vi "WW_Course_Wool_Parameter.vi"() -> (0 "strValveControlState":T1, 1 "strWaterLevel":T2, 2 "strTurnOnOff":T3, 3 "strAllTime":T4, 4 "mu16ArrayBubbleSoakState":u16[](array[numeric]), 5 "mu16ArrayHeating":u16[][](array[numeric]))   [LabVIEW 2011]
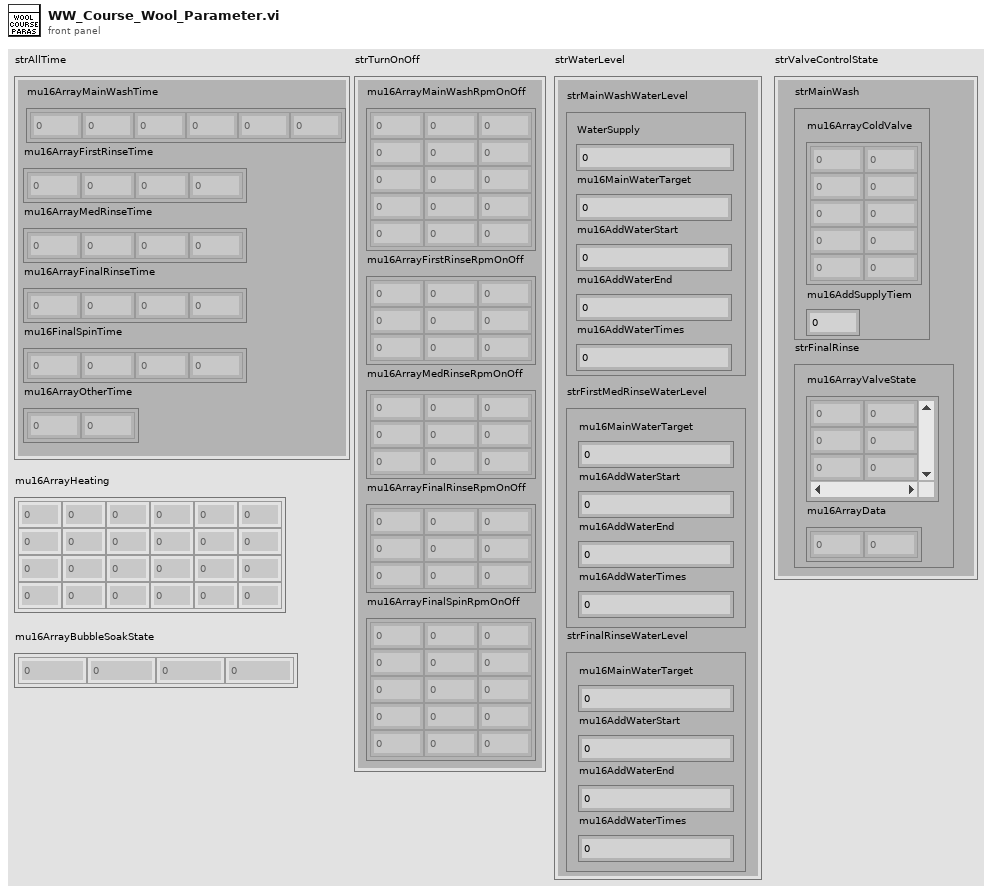
[diagram p1: front panel]
types:
  T1 = cluster{"strMainWash":cluster{"mu16ArrayColdValve":u8[][], "mu16AddSupplyTiem":u8}, "strFinalRinse":cluster{"mu16ArrayValveState":u8[][], "mu16ArrayData":u8[]}}
  T2 = cluster{"strMainWashWaterLevel":cluster{"WaterSupply":u16, "mu16MainWaterTarget":u16, "mu16AddWaterStart":u16, "mu16AddWaterEnd":u16, "mu16AddWaterTimes":u16}, "strFirstMedRinseWaterLevel":cluster{"mu16MainWaterTarget":u16, "mu16AddWaterStart":u16, "mu16AddWaterEnd":u16, "mu16AddWaterTimes":u16}, "strFinalRinseWaterLevel":cluster{"mu16MainWaterTarget":u16, "mu16AddWaterStart":u16, "mu16AddWaterEnd":u16, "mu16AddWaterTimes":u16}}
  T3 = cluster{"mu16ArrayMainWashRpmOnOff":u8[][], "mu16ArrayFirstRinseRpmOnOff":u8[][], "mu16ArrayMedRinseRpmOnOff":u8[][], "mu16ArrayFinalRinseRpmOnOff":u8[][], "mu16ArrayFinalSpinRpmOnOff":u16[][]}
  T4 = cluster{"mu16ArrayMainWashTime":u16[], "mu16ArrayFirstRinseTime":u16[], "mu16ArrayMedRinseTime":u16[], "mu16ArrayFinalRinseTime":u16[], "mu16FinalSpinTime":u16[], "mu16ArrayOtherTime":u16[]}
  T5 = enum8{"NULL", "Course", "eCotton", "Synthetics", "Wool", "Spin", "RinseSpin", "EcoDrumClean", "DarkGarment", "OutDoorCare", "BabyCare", "Delicates", "Bedding", "SuperEcoWash", "SuperSpeed"}
  T6 = cluster{"数组":u16[], "数组":u16[], "数组":u16[], "数组":u16[], "数组":u16[], "数组":u16[]}
  T7 = cluster{i32[][], i32[][], i32[][], i32[][], i32[][]}
  T8 = cluster{cluster{i32, i32, i32, i32, i32}, cluster{i32, i32, i32, i32}, cluster{"offset past number":i32, i32, i32, i32}}
  T9 = cluster{cluster{i32[][], i32}, cluster{i32[][], i32[]}}
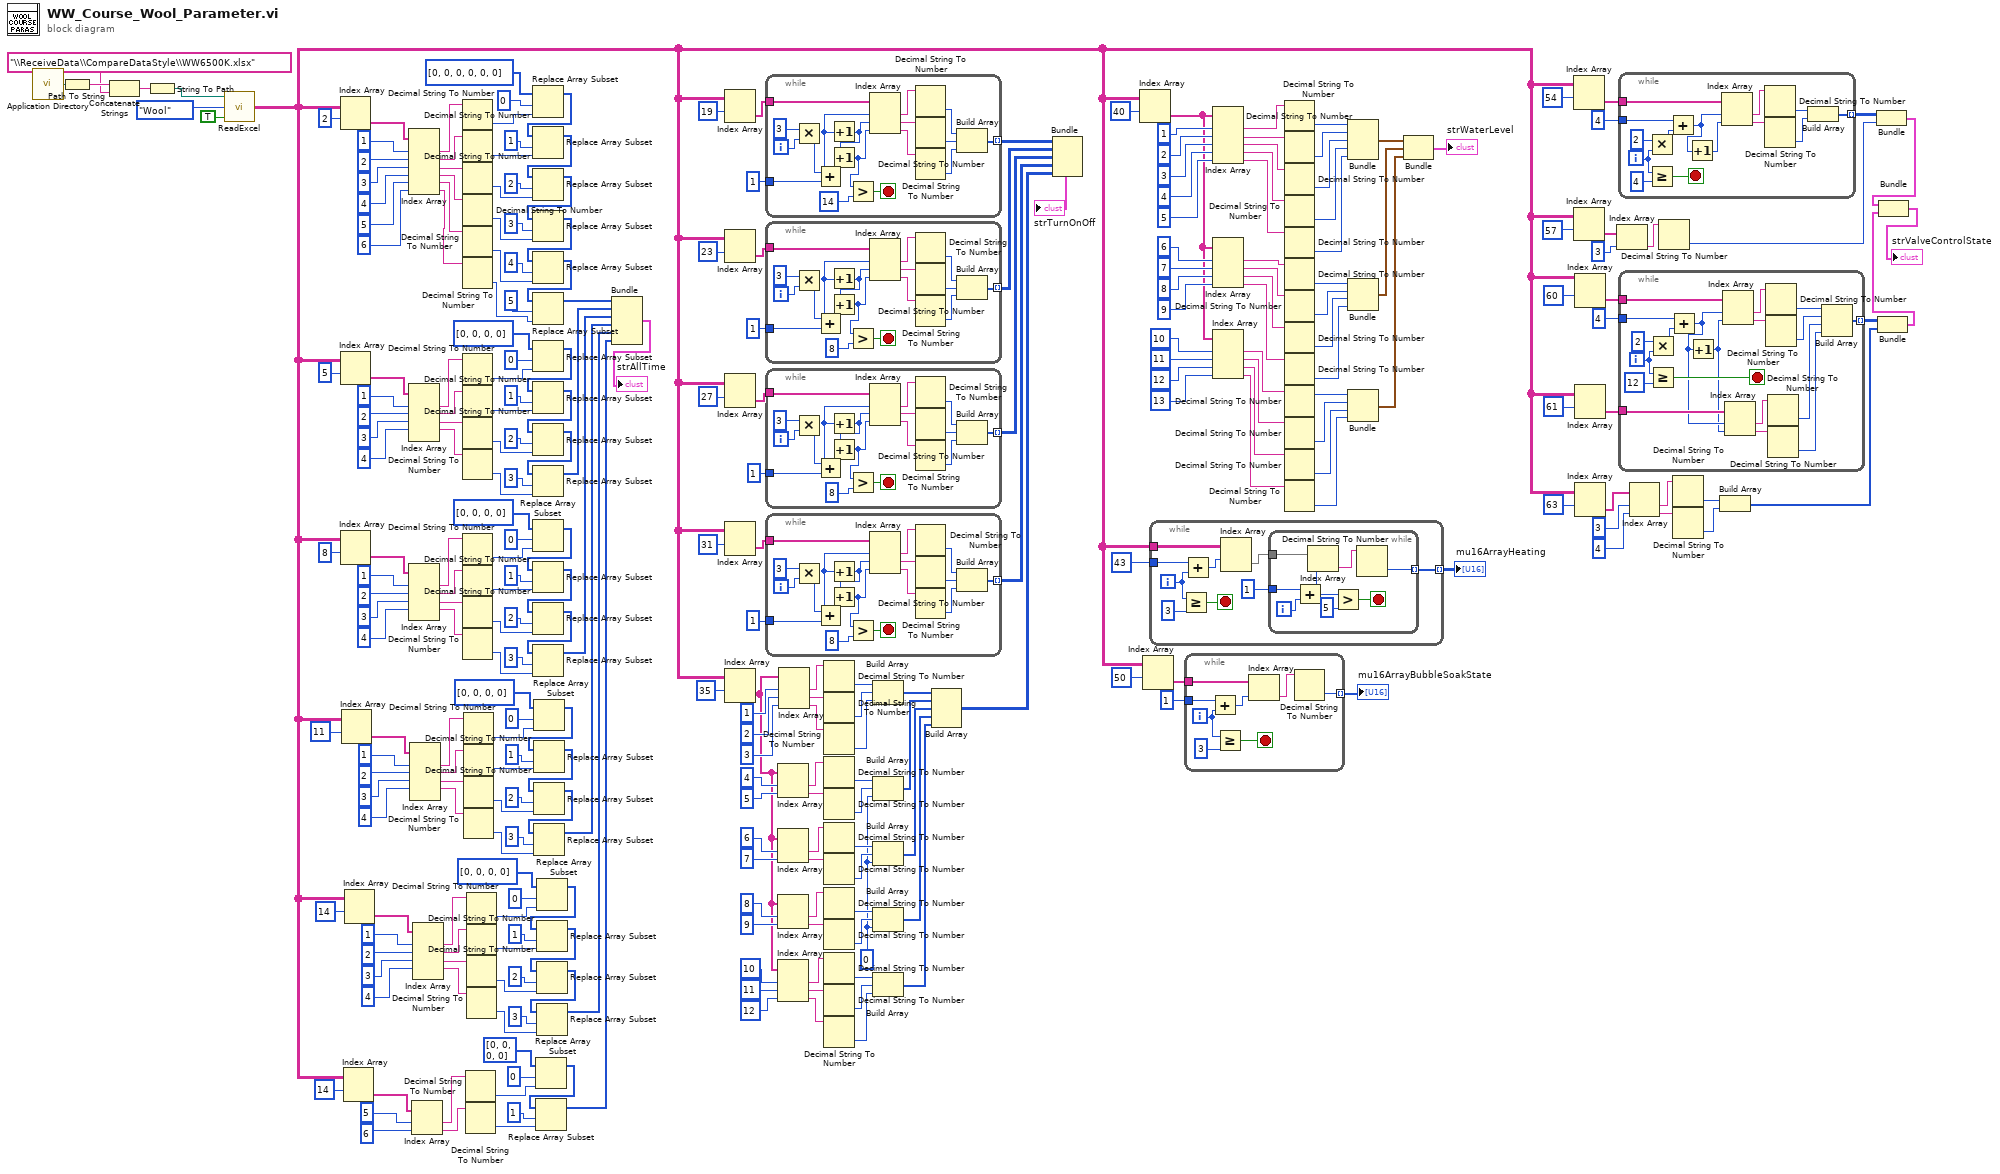
[diagram p0: block diagram]
diagram:
  w89 = 0 ("元素")
  n1 = call <vilib>:"Application Directory.vi"() -> ("Application Directory"=w143:path)
  n2 = Path To String(path=w143) -> (string=w142:string)
  n3 = Concatenate Strings(w142, "\\ReceiveData\\CompareDataStyle\\WW6500K.xlsx") -> (w140:string)
  n4 = String To Path(string=w140) -> (path=w139:path)
  n5 = call "ReadExcel.vi"("读出文本"=TRUE, "导出sheet位号"=T5."Wool" ("enumCourse"), "路径"=w139) -> ("EXCEL读取"=w12:string[][])
  n6 = Index Array(array=w12, index (row)=2 ("索引 (行)")) -> (element=w284:string[])  [unwired: 1 in]
  n7 = Index Array(array=w12, index (row)=5 ("索引 (行)")) -> (element=w257:string[])  [unwired: 1 in]
  n8 = Index Array(array=w12, index (row)=8 ("索引 (行)")) -> (element=w235:string[])  [unwired: 1 in]
  n9 = Index Array(array=w12, index (row)=11 ("索引 (行)")) -> (element=w213:string[])  [unwired: 1 in]
  n10 = Index Array(array=w12, index (row)=14 ("索引 (行)")) -> (element=w169:string[])  [unwired: 1 in]
  n11 = Index Array(array=w12, index (row)=14 ("索引 (行)")) -> (element=w191:string[])  [unwired: 1 in]
  n12 = Index Array(array=w284, index #1=1 ("索引"), index #2=2 ("索引"), index #3=3 ("索引"), index #4=4 ("索引"), index #5=5 ("索引"), index #6=6 ("索引")) -> (element #1=w278:string, element #2=w277:string, element #3=w276:string, element #4=w275:string, element #5=w274:string, element #6=w149:string)
  n13 = Index Array(array=w257, index #1=1 ("索引"), index #2=2 ("索引"), index #3=3 ("索引"), index #4=4 ("索引")) -> (element #1=w252:string, element #2=w251:string, element #3=w250:string, element #4=w249:string)  [unwired: 1 in, 1 out]
  n14 = Index Array(array=w235, index #1=1 ("索引"), index #2=2 ("索引"), index #3=3 ("索引"), index #4=4 ("索引")) -> (element #1=w230:string, element #2=w229:string, element #3=w228:string, element #4=w227:string)  [unwired: 1 in, 1 out]
  n15 = Index Array(array=w213, index #1=1 ("索引"), index #2=2 ("索引"), index #3=3 ("索引"), index #4=4 ("索引")) -> (element #1=w208:string, element #2=w207:string, element #3=w206:string, element #4=w205:string)  [unwired: 1 in, 1 out]
  n16 = Index Array(array=w169, index #1=5 ("索引"), index #2=6 ("索引")) -> (element #1=w166:string, element #2=w165:string)
  n17 = Index Array(array=w191, index #1=1 ("索引"), index #2=2 ("索引"), index #3=3 ("索引"), index #4=4 ("索引")) -> (element #1=w186:string, element #2=w185:string, element #3=w184:string, element #4=w183:string)  [unwired: 1 in, 1 out]
  n18 = Decimal String To Number(string=w278) -> (number=w272:i32)  [unwired: 2 in, 1 out]
  n19 = Decimal String To Number(string=w277) -> (number=w266:i32)  [unwired: 2 in, 1 out]
  n20 = Decimal String To Number(string=w276) -> (number=w265:i32)  [unwired: 2 in, 1 out]
  n21 = Decimal String To Number(string=w275) -> (number=w264:i32)  [unwired: 2 in, 1 out]
  n22 = Decimal String To Number(string=w274) -> (number=w263:i32)  [unwired: 2 in, 1 out]
  n23 = Decimal String To Number(string=w149) -> (number=w150:i32)  [unwired: 2 in, 1 out]
  n24 = Decimal String To Number(string=w252) -> (number=w247:i32)  [unwired: 2 in, 1 out]
  n25 = Decimal String To Number(string=w251) -> (number=w242:i32)  [unwired: 2 in, 1 out]
  n26 = Decimal String To Number(string=w250) -> (number=w241:i32)  [unwired: 2 in, 1 out]
  n27 = Decimal String To Number(string=w249) -> (number=w240:i32)  [unwired: 2 in, 1 out]
  n28 = Decimal String To Number(string=w230) -> (number=w225:i32)  [unwired: 2 in, 1 out]
  n29 = Decimal String To Number(string=w229) -> (number=w220:i32)  [unwired: 2 in, 1 out]
  n30 = Decimal String To Number(string=w228) -> (number=w219:i32)  [unwired: 2 in, 1 out]
  n31 = Decimal String To Number(string=w227) -> (number=w218:i32)  [unwired: 2 in, 1 out]
  n32 = Decimal String To Number(string=w208) -> (number=w203:i32)  [unwired: 2 in, 1 out]
  n33 = Decimal String To Number(string=w207) -> (number=w198:i32)  [unwired: 2 in, 1 out]
  n34 = Decimal String To Number(string=w206) -> (number=w197:i32)  [unwired: 2 in, 1 out]
  n35 = Decimal String To Number(string=w205) -> (number=w196:i32)  [unwired: 2 in, 1 out]
  n36 = Decimal String To Number(string=w166) -> (number=w163:i32)  [unwired: 2 in, 1 out]
  n37 = Decimal String To Number(string=w165) -> (number=w160:i32)  [unwired: 2 in, 1 out]
  n38 = Decimal String To Number(string=w186) -> (number=w181:i32)  [unwired: 2 in, 1 out]
  n39 = Decimal String To Number(string=w185) -> (number=w176:i32)  [unwired: 2 in, 1 out]
  n40 = Decimal String To Number(string=w184) -> (number=w175:i32)  [unwired: 2 in, 1 out]
  n41 = Decimal String To Number(string=w183) -> (number=w174:i32)  [unwired: 2 in, 1 out]
  n42 = Replace Array Subset(array=u16[] [0, 0, 0, 0, 0, 0] ("数组"), new element=w272, index=0 ("索引")) -> (w270:u16[])
  n43 = Replace Array Subset(array=w270, new element=w266, index=1 ("索引")) -> (w269:u16[])
  n44 = Replace Array Subset(array=w269, new element=w265, index=2 ("索引")) -> (w268:u16[])
  n45 = Replace Array Subset(array=w268, new element=w264, index=3 ("索引")) -> (w267:u16[])
  n46 = Replace Array Subset(array=w267, new element=w263, index=4 ("索引")) -> (w152:u16[])
  n47 = Replace Array Subset(array=w152, new element=w150, index=5 ("索引")) -> (w148:u16[])
  n48 = Replace Array Subset(array=u16[] [0, 0, 0, 0] ("数组"), new element=w247, index=0 ("索引")) -> (w245:u16[])
  n49 = Replace Array Subset(array=w245, new element=w242, index=1 ("索引")) -> (w244:u16[])
  n50 = Replace Array Subset(array=w244, new element=w241, index=2 ("索引")) -> (w243:u16[])
  n51 = Replace Array Subset(array=w243, new element=w240, index=3 ("索引")) -> (w158:u16[])
  n52 = Replace Array Subset(array=u16[] [0, 0, 0, 0] ("数组"), new element=w225, index=0 ("索引")) -> (w223:u16[])
  n53 = Replace Array Subset(array=w223, new element=w220, index=1 ("索引")) -> (w222:u16[])
  n54 = Replace Array Subset(array=w222, new element=w219, index=2 ("索引")) -> (w221:u16[])
  n55 = Replace Array Subset(array=w221, new element=w218, index=3 ("索引")) -> (w157:u16[])
  n56 = Replace Array Subset(array=u16[] [0, 0, 0, 0] ("数组"), new element=w203, index=0 ("索引")) -> (w201:u16[])
  n57 = Replace Array Subset(array=w201, new element=w198, index=1 ("索引")) -> (w200:u16[])
  n58 = Replace Array Subset(array=w200, new element=w197, index=2 ("索引")) -> (w199:u16[])
  n59 = Replace Array Subset(array=w199, new element=w196, index=3 ("索引")) -> (w156:u16[])
  n60 = Replace Array Subset(array=u16[] [0, 0, 0, 0] ("数组"), new element=w163, index=0 ("索引")) -> (w161:u16[])
  n61 = Replace Array Subset(array=w161, new element=w160, index=1 ("索引")) -> (w154:u16[])
  n62 = Replace Array Subset(array=u16[] [0, 0, 0, 0] ("数组"), new element=w181, index=0 ("索引")) -> (w179:u16[])
  n63 = Replace Array Subset(array=w179, new element=w176, index=1 ("索引")) -> (w178:u16[])
  n64 = Replace Array Subset(array=w178, new element=w175, index=2 ("索引")) -> (w177:u16[])
  n65 = Replace Array Subset(array=w177, new element=w174, index=3 ("索引")) -> (w155:u16[])
  n66 = Bundle("数组"=w148, "数组"=w158, "数组"=w157, "数组"=w156, "数组"=w155, "数组"=w154) -> (→"strAllTime":T6)  [unwired: 1 in]
  n67 = Index Array(array=w12, index (row)=19 ("索引 (行)")) -> (element=w145:string[])  [unwired: 1 in]
  n68 = Index Array(array=w12, index (row)=23 ("索引 (行)")) -> (element=w135:string[])  [unwired: 1 in]
  n69 = Index Array(array=w12, index (row)=27 ("索引 (行)")) -> (element=w131:string[])  [unwired: 1 in]
  n70 = Index Array(array=w12, index (row)=31 ("索引 (行)")) -> (element=w127:string[])  [unwired: 1 in]
  n71 = Index Array(array=w12, index (row)=35 ("索引 (行)")) -> (element=w94:string[])  [unwired: 1 in]
  n72 = while {
    tunnel: w145 -> [w304]
    tunnel: 1 -> [w303]
    tunnel: [w290] -> w138 mode=indexing
    i -> [w297]
    stop <- w301 stop-if-true
    n73 = Multiply(x=3 ("y"), y=w297) -> (x*y=w299:i32)
    n74 = Add(x=w299, y=w303) -> (x+y=w294:i32)
    n75 = Increment(x=w294) -> (x+1=w289:i32)
    n76 = Increment(x=w289) -> (x+1=w288:i32)
    n77 = Greater?(x=w288, y=14) -> (0:w301:bool)
    n78 = Index Array(array=w304, index #1=w294, index #2=w289, index #3=w288) -> (element #1=w300:string, element #2=w296:string, element #3=w295:string)
    n79 = Decimal String To Number(string=w300) -> (number=w292:i32)  [unwired: 2 in, 1 out]
    n80 = Decimal String To Number(string=w296) -> (number=w293:i32)  [unwired: 2 in, 1 out]
    n81 = Decimal String To Number(string=w295) -> (number=w291:i32)  [unwired: 2 in, 1 out]
    n82 = Build Array(w292, w293, w291) -> (w290:i32[])
  }
  n83 = while {
    tunnel: w135 -> [w321]
    tunnel: 1 -> [w320]
    tunnel: [w307] -> w134 mode=indexing
    i -> [w314]
    stop <- w318 stop-if-true
    n84 = Multiply(x=3 ("y"), y=w314) -> (x*y=w316:i32)
    n85 = Add(x=w316, y=w320) -> (x+y=w311:i32)
    n86 = Increment(x=w311) -> (x+1=w306:i32)
    n87 = Increment(x=w306) -> (x+1=w305:i32)
    n88 = Greater?(x=w305, y=8) -> (0:w318:bool)
    n89 = Index Array(array=w321, index #1=w311, index #2=w306, index #3=w305) -> (element #1=w317:string, element #2=w313:string, element #3=w312:string)
    n90 = Decimal String To Number(string=w317) -> (number=w309:i32)  [unwired: 2 in, 1 out]
    n91 = Decimal String To Number(string=w313) -> (number=w310:i32)  [unwired: 2 in, 1 out]
    n92 = Decimal String To Number(string=w312) -> (number=w308:i32)  [unwired: 2 in, 1 out]
    n93 = Build Array(w309, w310, w308) -> (w307:i32[])
  }
  n94 = while {
    tunnel: w131 -> [w338]
    tunnel: 1 -> [w337]
    tunnel: [w324] -> w130 mode=indexing
    i -> [w331]
    stop <- w335 stop-if-true
    n95 = Multiply(x=3 ("y"), y=w331) -> (x*y=w333:i32)
    n96 = Add(x=w333, y=w337) -> (x+y=w328:i32)
    n97 = Increment(x=w328) -> (x+1=w323:i32)
    n98 = Increment(x=w323) -> (x+1=w322:i32)
    n99 = Greater?(x=w322, y=8) -> (0:w335:bool)
    n100 = Index Array(array=w338, index #1=w328, index #2=w323, index #3=w322) -> (element #1=w334:string, element #2=w330:string, element #3=w329:string)
    n101 = Decimal String To Number(string=w334) -> (number=w326:i32)  [unwired: 2 in, 1 out]
    n102 = Decimal String To Number(string=w330) -> (number=w327:i32)  [unwired: 2 in, 1 out]
    n103 = Decimal String To Number(string=w329) -> (number=w325:i32)  [unwired: 2 in, 1 out]
    n104 = Build Array(w326, w327, w325) -> (w324:i32[])
  }
  n105 = while {
    tunnel: w127 -> [w355]
    tunnel: 1 -> [w354]
    tunnel: [w341] -> w126 mode=indexing
    i -> [w348]
    stop <- w352 stop-if-true
    n106 = Multiply(x=3 ("y"), y=w348) -> (x*y=w350:i32)
    n107 = Add(x=w350, y=w354) -> (x+y=w345:i32)
    n108 = Increment(x=w345) -> (x+1=w340:i32)
    n109 = Increment(x=w340) -> (x+1=w339:i32)
    n110 = Greater?(x=w339, y=8) -> (0:w352:bool)
    n111 = Index Array(array=w355, index #1=w345, index #2=w340, index #3=w339) -> (element #1=w351:string, element #2=w347:string, element #3=w346:string)
    n112 = Decimal String To Number(string=w351) -> (number=w343:i32)  [unwired: 2 in, 1 out]
    n113 = Decimal String To Number(string=w347) -> (number=w344:i32)  [unwired: 2 in, 1 out]
    n114 = Decimal String To Number(string=w346) -> (number=w342:i32)  [unwired: 2 in, 1 out]
    n115 = Build Array(w343, w344, w342) -> (w341:i32[])
  }
  n116 = Index Array(array=w94, index #1=4, index #2=5) -> (element #1=w113:string, element #2=w112:string)
  n117 = Index Array(array=w94, index #1=6, index #2=7) -> (element #1=w35:string, element #2=w107:string)
  n118 = Index Array(array=w94, index #1=8, index #2=9) -> (element #1=w34:string, element #2=w102:string)
  n119 = Index Array(array=w94, index #1=10, index #2=11, index #3=12) -> (element #1=w92:string, element #2=w97:string, element #3=w91:string)
  n120 = Index Array(array=w94, index #1=1, index #2=2, index #3=3) -> (element #1=w121:string, element #2=w120:string, element #3=w119:string)
  n121 = Decimal String To Number(string=w121) -> (number=w118:i32)  [unwired: 2 in, 1 out]
  n122 = Decimal String To Number(string=w120) -> (number=w117:i32)  [unwired: 2 in, 1 out]
  n123 = Decimal String To Number(string=w119) -> (number=w116:i32)  [unwired: 2 in, 1 out]
  n124 = Decimal String To Number(string=w113) -> (number=w111:i32)  [unwired: 2 in, 1 out]
  n125 = Decimal String To Number(string=w112) -> (number=w110:i32)  [unwired: 2 in, 1 out]
  n126 = Decimal String To Number(string=w35) -> (number=w106:i32)  [unwired: 2 in, 1 out]
  n127 = Decimal String To Number(string=w107) -> (number=w105:i32)  [unwired: 2 in, 1 out]
  n128 = Decimal String To Number(string=w34) -> (number=w101:i32)  [unwired: 2 in, 1 out]
  n129 = Decimal String To Number(string=w102) -> (number=w100:i32)  [unwired: 2 in, 1 out]
  n130 = Decimal String To Number(string=w92) -> (number=w96:i32)  [unwired: 2 in, 1 out]
  n131 = Decimal String To Number(string=w97) -> (number=w95:i32)  [unwired: 2 in, 1 out]
  n132 = Decimal String To Number(string=w91) -> (number=w90:i32)  [unwired: 2 in, 1 out]
  n133 = Build Array(w118, w117, w116) -> (w88:i32[])
  n134 = Build Array(w111, w110, w89) -> (w87:i32[])
  n135 = Build Array(w106, w105, w89) -> (w86:i32[])
  n136 = Build Array(w101, w100, w89) -> (w85:i32[])
  n137 = Build Array(w96, w95, w90) -> (w84:i32[])
  n138 = Build Array(w88, w87, w86, w85, w84) -> (w83:i32[][])
  n139 = Bundle(w138, w134, w130, w126, w83) -> (→"strTurnOnOff":T7)  [unwired: 1 in]
  n140 = Index Array(array=w12, index (row)=40 ("索引 (行)")) -> (element=w67:string[])  [unwired: 1 in]
  n141 = Index Array(array=w12, index (row)=50 ("索引 (行)")) -> (element=w31:string[])  [unwired: 1 in]
  n142 = while {
    tunnel: w12 -> [w364]
    tunnel: 43 ("索引 (行)") -> [w363]
    tunnel: [w360] -> w33 mode=indexing
    i -> [w356]
    stop <- w358 stop-if-true
    n143 = Greater Or Equal?(x=w356, y=3) -> (x >= y?=w358:bool)
    n144 = Add(x=w363, y=w356) -> (x+y=w357:i32)
    n145 = Index Array(array=w364, index (row)=w357) -> (element=w362:string[])  [unwired: 1 in]
    n146 = while {
      tunnel: w362 -> [w370]
      tunnel: 1 ("索引") -> [w372]
      tunnel: [w365] -> w360 mode=indexing
      i -> [w371]
      stop <- w367 stop-if-true
      n147 = Add(x=w372, y=w371) -> (x+y=w369:i32)
      n148 = Index Array(array=w370, index=w369) -> (element=w366:string)
      n149 = Greater?(x=w369, y=5) -> (0:w367:bool)
      n150 = Decimal String To Number(string=w366) -> (number=w365:i32)  [unwired: 2 in, 1 out]
    }
  }
  "mu16ArrayHeating" <- w33
  n151 = while {
    tunnel: w31 -> [w378]
    tunnel: 1 ("y") -> [w380]
    tunnel: [w376] -> w29 mode=indexing
    i -> [w374]
    stop <- w373 stop-if-true
    n152 = Add(x=w380, y=w374) -> (x+y=w379:i32)
    n153 = Greater Or Equal?(x=w374, y=3) -> (x >= y?=w373:bool)
    n154 = Index Array(array=w378, index=w379) -> (element=w377:string)
    n155 = Decimal String To Number(string=w377) -> (number=w376:i32)  [unwired: 2 in, 1 out]
  }
  "mu16ArrayBubbleSoakState" <- w29
  n156 = Index Array(array=w67, index #1=1 ("索引"), index #2=2 ("索引"), index #3=3 ("索引"), index #4=4 ("索引"), index #5=5 ("索引")) -> (element #1=w63:string, element #2=w62:string, element #3=w61:string, element #4=w60:string, element #5=w59:string)
  n157 = Index Array(array=w67, index #1=6 ("索引"), index #2=7 ("索引"), index #3=8 ("索引"), index #4=9 ("索引")) -> (element #1=w53:string, element #2=w52:string, element #3=w51:string, element #4=w50:string)
  n158 = Index Array(array=w67, index #1=10 ("索引"), index #2=11 ("索引"), index #3=12 ("索引"), index #4=13 ("索引")) -> (element #1=w45:string, element #2=w44:string, element #3=w43:string, element #4=w42:string)
  n159 = Decimal String To Number(string=w63) -> (number=w58:i32)  [unwired: 2 in, 1 out]
  n160 = Decimal String To Number(string=w62) -> (number=w57:i32)  [unwired: 2 in, 1 out]
  n161 = Decimal String To Number(string=w61) -> (number=w56:i32)  [unwired: 2 in, 1 out]
  n162 = Decimal String To Number(string=w60) -> (number=w55:i32)  [unwired: 2 in, 1 out]
  n163 = Decimal String To Number(string=w59) -> (number=w54:i32)  [unwired: 2 in, 1 out]
  n164 = Decimal String To Number(string=w53) -> (number=w49:i32)  [unwired: 2 in, 1 out]
  n165 = Decimal String To Number(string=w52) -> (number=w48:i32)  [unwired: 2 in, 1 out]
  n166 = Decimal String To Number(string=w51) -> (number=w47:i32)  [unwired: 2 in, 1 out]
  n167 = Decimal String To Number(string=w50) -> (number=w46:i32)  [unwired: 2 in, 1 out]
  n168 = Decimal String To Number(string=w45) -> (offset past number=w41:i32)  [unwired: 2 in, 1 out]
  n169 = Decimal String To Number(string=w44) -> (number=w40:i32)  [unwired: 2 in, 1 out]
  n170 = Decimal String To Number(string=w43) -> (number=w39:i32)  [unwired: 2 in, 1 out]
  n171 = Decimal String To Number(string=w42) -> (number=w38:i32)  [unwired: 2 in, 1 out]
  n172 = Bundle(w58, w57, w56, w55, w54) -> (w66:cluster{i32, i32, i32, i32, i32})  [unwired: 1 in]
  n173 = Bundle(w49, w48, w47, w46) -> (w65:cluster{i32, i32, i32, i32})  [unwired: 1 in]
  n174 = Bundle("offset past number"=w41, w40, w39, w38) -> (w64:cluster{"offset past number":i32, i32, i32, i32})  [unwired: 1 in]
  n175 = Bundle(w66, w65, w64) -> (→"strWaterLevel":T8)  [unwired: 1 in]
  n176 = Index Array(array=w12, index (row)=54 ("索引 (行)")) -> (element=w27:string[])  [unwired: 1 in]
  n177 = Index Array(array=w12, index (row)=57 ("索引 (行)")) -> (element=w23:string[])  [unwired: 1 in]
  n178 = Index Array(array=w12, index (row)=60 ("索引 (行)")) -> (element=w18:string[])  [unwired: 1 in]
  n179 = Index Array(array=w12, index (row)=61 ("索引 (行)")) -> (element=w15:string[])  [unwired: 1 in]
  n180 = Index Array(array=w12, index (row)=63 ("索引 (行)")) -> (element=w10:string[])  [unwired: 1 in]
  n181 = Index Array(array=w23, index=3 ("索引 (行)")) -> (element=w21:string)
  n182 = while {
    tunnel: w27 -> [w391]
    tunnel: 4 -> [w392]
    tunnel: [w385] -> w25 mode=indexing
    i -> [w384]
    stop <- w382 stop-if-true
    n183 = Multiply(x=2 ("y"), y=w384) -> (x*y=w393:i32)
    n184 = Greater Or Equal?(x=w384, y=4) -> (x >= y?=w382:bool)
    n185 = Add(x=w392, y=w393) -> (x+y=w390:i32)
    n186 = Increment(x=w390) -> (x+1=w381:i32)
    n187 = Index Array(array=w391, index #1=w390, index #2=w381) -> (element #1=w389:string, element #2=w388:string)
    n188 = Decimal String To Number(string=w389) -> (number=w387:i32)  [unwired: 2 in, 1 out]
    n189 = Decimal String To Number(string=w388) -> (number=w386:i32)  [unwired: 2 in, 1 out]
    n190 = Build Array(w387, w386) -> (w385:i32[])
  }
  n191 = while {
    tunnel: w18 -> [w410]
    tunnel: 4 -> [w411]
    tunnel: [w405] -> w14 mode=indexing
    tunnel: w15 -> [w399]
    i -> [w404]
    stop <- w402 stop-if-true
    n192 = Multiply(x=2 ("y"), y=w404) -> (x*y=w412:i32)
    n193 = Greater Or Equal?(x=w404, y=12) -> (x >= y?=w402:bool)
    n194 = Add(x=w411, y=w412) -> (x+y=w398:i32)
    n195 = Increment(x=w398) -> (x+1=w397:i32)
    n196 = Index Array(array=w410, index #1=w398, index #2=w397) -> (element #1=w409:string, element #2=w408:string)
    n197 = Index Array(array=w399, index #1=w398, index #2=w397) -> (element #1=w401:string, element #2=w400:string)
    n198 = Decimal String To Number(string=w409) -> (number=w407:i32)  [unwired: 2 in, 1 out]
    n199 = Decimal String To Number(string=w408) -> (number=w406:i32)  [unwired: 2 in, 1 out]
    n200 = Decimal String To Number(string=w401) -> (number=w396:i32)  [unwired: 2 in, 1 out]
    n201 = Decimal String To Number(string=w400) -> (number=w395:i32)  [unwired: 2 in, 1 out]
    n202 = Build Array(w407, w406, w396, w395) -> (w405:i32[])
  }
  n203 = Index Array(array=w10, index #1=3, index #2=4) -> (element #1=w7:string, element #2=w11:string)
  n204 = Decimal String To Number(string=w21) -> (number=w20:i32)  [unwired: 2 in, 1 out]
  n205 = Decimal String To Number(string=w7) -> (number=w6:i32)  [unwired: 2 in, 1 out]
  n206 = Decimal String To Number(string=w11) -> (number=w5:i32)  [unwired: 2 in, 1 out]
  n207 = Build Array(w6, w5) -> (w4:i32[])
  n208 = Bundle(w25, w20) -> (w3:cluster{i32[][], i32})  [unwired: 1 in]
  n209 = Bundle(w14, w4) -> (w2:cluster{i32[][], i32[]})  [unwired: 1 in]
  n210 = Bundle(w3, w2) -> (→"strValveControlState":T9)  [unwired: 1 in]
